vi "FTW-ProjectItemManager-AddToRemoveTransaction.vi"(0 "Project Item Manager":refnum<class "FTW-ProjectItemManager.lvclass">, 5 "Regex Matches to Remove":string, 7 "Force Literal Match?":bool, 11 "error in":errorcluster) -> (4 "Project Item Manager out":refnum<class "FTW-ProjectItemManager.lvclass">, 15 "error out":errorcluster)   [LabVIEW 2012, in "FTW-ProjectItemManager.lvclass"]
uses:
  FTW-ProjectItemManager.lvclass
  FTW-ProjectItemManager.lvclass/FTW-ProjectItemManager.ctl
panel:
  # "Inputs"
  # "Outputs"
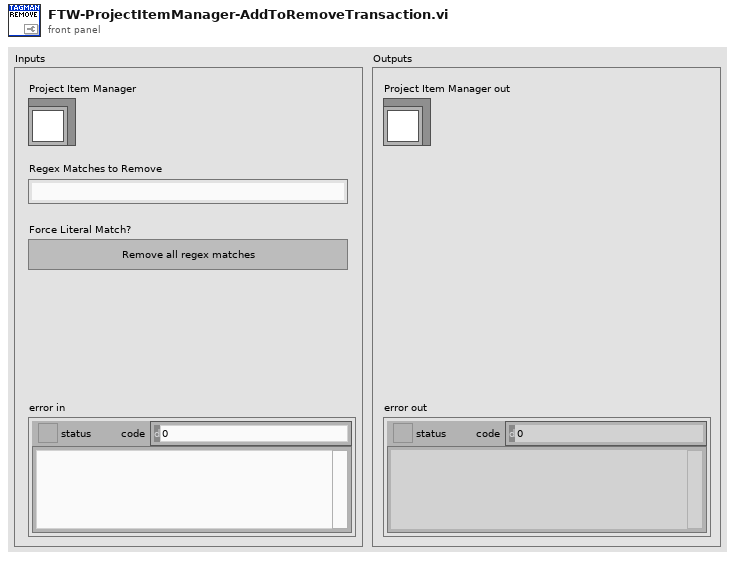
[diagram p1: front panel]
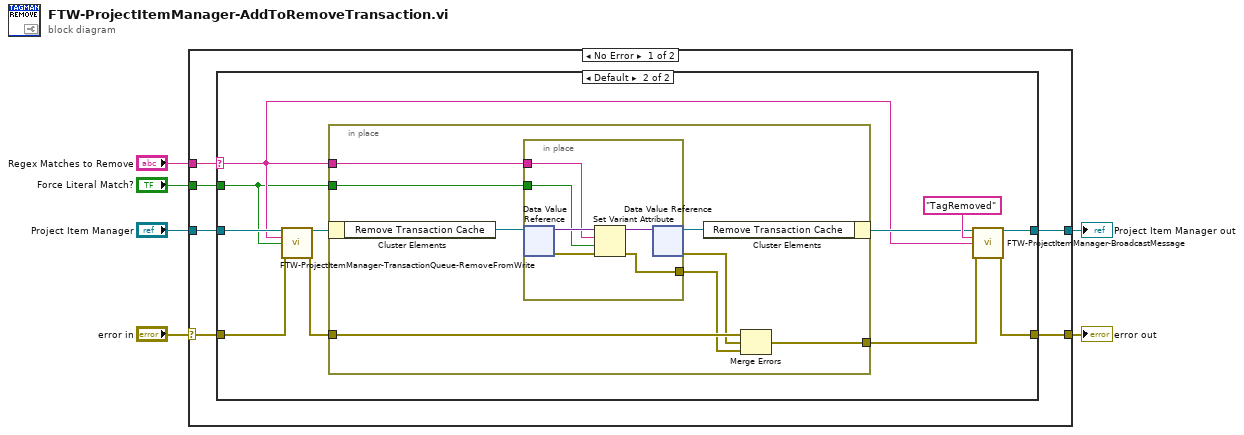
[diagram p0: block diagram]
diagram:
  n1 = case shown="No Error" "error in" {
    selector: "error in" -> [w12 w41]
    tunnel: [w11 w41] -> w6
    tunnel: [w9 w40] -> w4
    tunnel: "Project Item Manager" -> [w10 w40]
    tunnel: "Regex Matches to Remove" -> [w8 _]
    tunnel: "Force Literal Match?" -> [w7 _]
    frame No Error {
      n2 = case shown="Default" w8 {
        selector: w8 -> [_ w16]
        tunnel: w12 -> [w13 w18]
        tunnel: [w13 w22] -> w11
        tunnel: w10 -> [w14 w20]
        tunnel: [w14 w23] -> w9
        tunnel: w7 -> [_ w15]
        frame "" {
        }
        frame Default {
          n3 = call "FTW-ProjectItemManager-TransactionQueue-RemoveFromWrite.vi"("Project Item Manager"=w20, "Tag Regex to Match"=w16, "Force Literal Match?"=w15, "error in"=w18) -> ("Project Item Manager out"=w19:refnum<class "FTW-ProjectItemManager.lvclass">, "error out"=w17:errorcluster)  [unwired: 10 in]
          n4 = in-place {
            in-place-border: [w31] -> w21
            in-place-border: w16 -> [w30]
            in-place-border: w15 -> [w29]
            in-place-border: w17 -> [w28]
            n5 = in-place-cluster #1(w19) -> ("Remove Transaction Cache"=w33:refnum<data-value>)
            n6 = in-place {
              in-place-border: [w39] -> w26
              in-place-border: w30 -> [w35]
              in-place-border: w29 -> [w34]
              n7 = in-place-dvr #2(w33) -> (w38:variant, w36:errorcluster)
              n8 = Set Variant Attribute(Variant=w38, name=w35, value=w34, error in=w36) -> (Variant out=w37:variant, error out=w39:errorcluster)  [unwired: 1 out]
              n9 = in-place-dvr #2(w37) -> (w32:refnum<data-value>, w27:errorcluster)
            }
            n10 = in-place-cluster #1("Remove Transaction Cache"=w32) -> (w24:refnum<class "FTW-ProjectItemManager.lvclass">)
            n11 = Merge Errors(w28, w27, w26) -> (w31:errorcluster)
          }
          n12 = call "FTW-ProjectItemManager-BroadcastMessage.vi"("Project Item Manager"=w24, "Action Performed"="TagRemoved", "Payload"=w16, "error in"=w21) -> ("Project Item Manager out"=w23:refnum<class "FTW-ProjectItemManager.lvclass">, "error out"=w22:errorcluster)  [unwired: 10 in]
        }
      }
    }
    frame Error {
    }
  }
  "error out" <- w6
  "Project Item Manager out" <- w4
